vi "Unescape percent-encoding.vi"(2 "percent-encoded string":string, 3 "error in (no error)":errorcluster, 4 "safe?":bool) -> (9 "decoded string":string, 10 "error out":errorcluster)   [LabVIEW 2020, in "NI_WFCN.lvlib"]
doc: "Unescape a URL percent-encoding from the specified string."
uses:
  <vilib>/net/WFCN/NI_WFCN.lvlib
panel:
  in  "invalid fmt text":string="Invalid percent-encoding in: "
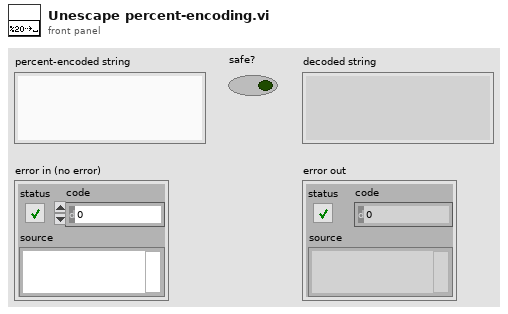
[diagram p1: front panel]
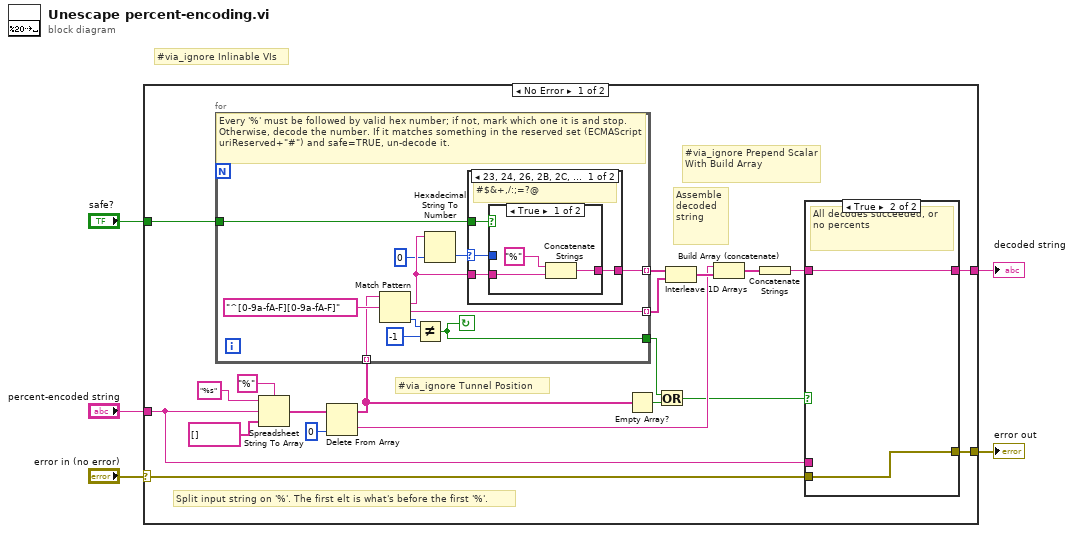
[diagram p0: block diagram]
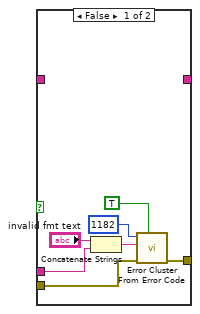
[diagram p2: hidden frame]
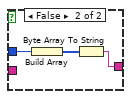
[diagram p3: hidden frame]
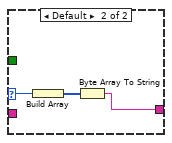
[diagram p4: hidden frame]
diagram:
  # "#via_ignore Inlinable VIs"
  n1 = case shown="No Error" "error in (no error)" {
    selector: "error in (no error)" -> [w6 w59]
    tunnel: "percent-encoded string" -> [w25 _]
    tunnel: [w24 _] -> w4
    tunnel: [w23 w59] -> w2
    tunnel: "safe?" -> [w7 _]
    frame No Error {
      # "#via_ignore Prepend Scalar With Build Array"
      # "#via_ignore Tunnel Position"
      # "Split input string on '%'. The first elt is what's before the first '%'."
      # "Assemble decoded string"
      n2 = Spreadsheet String To Array(delimiter (Tab)="%", format string="%s", spreadsheet string=w25, array type (2D Dbl)=string[] []) -> (array=w19:string[])
      n3 = Delete From Array(array=w19, index=0) -> (deleted portion=w15:string, array with subset deleted=w8:string[])  [unwired: 1 in]
      n4 = for {
        tunnel: w8 -> [w43] mode=indexing
        tunnel: w7 -> [w35]
        tunnel: [w42] -> w17 mode=indexing
        tunnel: [w41] -> w11 mode=indexing
        tunnel: [w37] -> w12
        stop <- w37 continue-if-true
        # "Every '%' must be followed by valid hex number; if not, mark which one it is and stop. Otherwise, decode the number. If it matches something in the reserved set (ECMAScript uriReserved+\"#\") and safe=TRUE, un-decode it."
        n5 = Match Pattern(string=w43, regular expression="^[0-9a-fA-F][0-9a-fA-F]") -> (match substring=w44:string, after substring=w41:string, offset past match=w39:i32)  [unwired: 1 in, 1 out]
        n6 = Not Equal?(x=w39, y=-1) -> (x != y?=w37:bool)
        n7 = Hexadecimal String To Number(string=w44, default (0uL)=u8 0 ("default (0 U32)")) -> (number=w36:u8)  [unwired: 1 in, 1 out]
        n8 = case shown="23, 24, 26, 2B, 2C, 2F, 3A, 3B, 3D, 3F, 40" w36 {
          selector: w36 -> [w47 w57]
          tunnel: w44 -> [w49 _]
          tunnel: [w48 w56] -> w42
          tunnel: w35 -> [w46 _]
          frame 35, 36, 38, 43, 44, 47, 58, 59, 61, 63, 64 {
            # "#$&+,/:;=?@"
            n9 = case shown="True" w46 {
              tunnel: w47 -> [_ w55]
              tunnel: [w51 w53] -> w48
              tunnel: w49 -> [w52 _]
              frame True {
                n10 = Concatenate Strings("%" ("string"), w52) -> (w51:string)
              }
              frame False {
                n11 = Build Array(w55) -> (w54:u8[])
                n12 = Byte Array To String(unsigned byte array=w54) -> (string=w53:string)
              }
            }
          }
          frame Default {
            n13 = Build Array(w57) -> (w58:u8[])
            n14 = Byte Array To String(unsigned byte array=w58) -> (string=w56:string)
          }
        }
      }
      n15 = Empty Array?(array=w8) -> (empty?=w10:bool)
      n16 = Or(x=w12, y=w10) -> (x .or. y?=w9:bool)
      n17 = Interleave 1D Arrays(w17, w11) -> (w16:string[])
      n18 = Build Array (concatenate)(w15, w16) -> (w14:string[])
      n19 = Concatenate Strings(w14) -> (w13:string)
      n20 = case shown="True" w9 {
        tunnel: w13 -> [_ w34]
        tunnel: [_ w34] -> w24
        tunnel: [w31 w33] -> w23
        tunnel: w25 -> [w28 _]
        tunnel: w6 -> [w26 w33]
        frame False {
          n21 = Concatenate Strings("invalid fmt text", w28) -> (w29:string)
          n22 = call <vilib>:"Error Cluster From Error Code.vi"("show call chain? (False)"=TRUE, "error in (no error)"=w26, "error message (\"\")"=w29, "error code (0)"=1182) -> ("error out"=w31:errorcluster)  [unwired: 5 in]
        }
        frame True {
          # "All decodes succeeded, or no percents"
        }
      }
    }
    frame Error {
    }
  }
  "decoded string" <- w4
  "error out" <- w2
